vi "CalcVectors.vi"(8 "In/out":dbl, 9 "Up/down":dbl, 10 "Shoulder Degrees":dbl, 11 "Elbow Degrees":dbl) -> (2 "Shoulder Power":dbl, 3 "Elbow power":dbl)   [LabVIEW 2018]
panel:
  out "Theta C 2":dbl
  out "Theta b 2":dbl
  out "sin(b) 2":dbl
  out "sin(c) 2":dbl
  out "sin(b)":dbl
  out "sin(c)":dbl
  out "Theta C":dbl
  out "Theta b":dbl
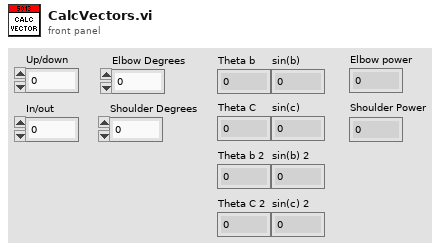
[diagram p1: front panel]
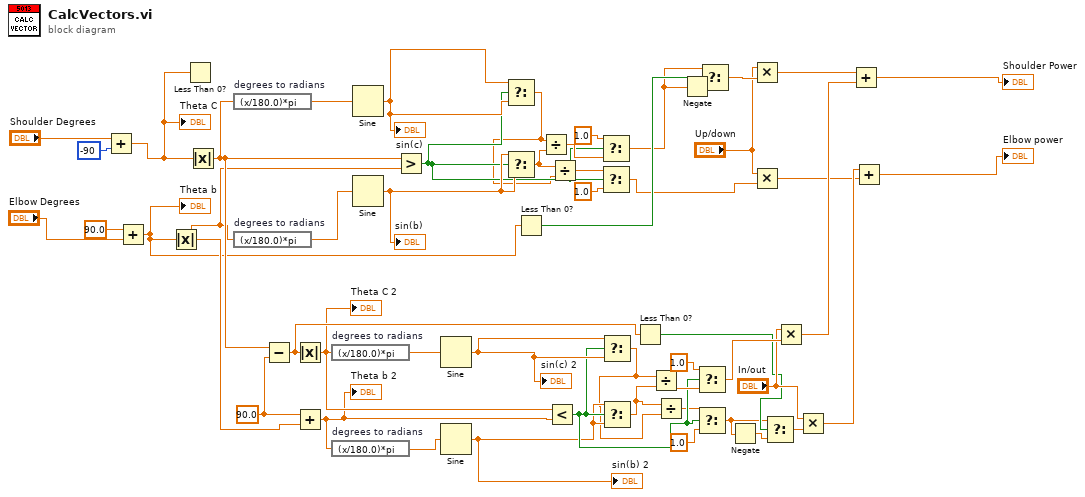
[diagram p0: block diagram]
diagram:
  w26 = 90.0 ("x")
  n1 = Add(x="Shoulder Degrees", y=-90) -> (x+y=w49:dbl)
  "Theta C" <- w49
  n2 = Add(x=90.0, y="Elbow Degrees") -> (x+y=w20:dbl)
  "Theta b" <- w20
  n3 = Absolute Value(x=w20) -> (abs(x)=w45:dbl)
  n4 = Less Than 0?(x=w49) -> ()  [unwired: 1 out]
  n5 = Absolute Value(x=w49) -> (abs(x)=w46:dbl)
  n6 = expression code="(x/180.0)*pi" "degrees to radians"(w46) -> (w43:dbl)
  n7 = expression code="(x/180.0)*pi" "degrees to radians"(w45) -> (w42:dbl)
  n8 = Subtract(x=w46, y=w26) -> (x-y=w25:dbl)
  n9 = Absolute Value(x=w25) -> (abs(x)=w18:dbl)
  "Theta C 2" <- w18
  n10 = Add(x=w26, y=w45) -> (x+y=w17:dbl)
  "Theta b 2" <- w17
  n11 = expression code="(x/180.0)*pi" "degrees to radians"(w18) -> (w33:dbl)
  n12 = expression code="(x/180.0)*pi" "degrees to radians"(w17) -> (w32:dbl)
  n13 = Sine(x=w43) -> (sin(x)=w41:dbl)
  "sin(c)" <- w41
  n14 = Sine(x=w42) -> (sin(x)=w40:dbl)
  "sin(b)" <- w40
  n15 = Greater?(x=w46, y=w45) -> (0:w34:bool)
  n16 = Sine(x=w33) -> (sin(x)=w31:dbl)
  "sin(c) 2" <- w31
  n17 = Sine(x=w32) -> (sin(x)=w21:dbl)
  "sin(b) 2" <- w21
  n18 = Select(t=w41, s=w34, f=w41) -> (s? t:f=w14:dbl)
  n19 = Select(t=w40, s=w34, f=w40) -> (s? t:f=w15:dbl)
  n20 = Less Than 0?(x=w20) -> (x < 0?=w13:bool)
  n21 = Divide(x=w14, y=w15) -> (x/y=w38:dbl)
  n22 = Less?(x=w18, y=w17) -> (x < y?=w24:bool)
  n23 = Divide(x=w15, y=w14) -> (x/y=w16:dbl)
  n24 = Select(t=1.0, s=w34, f=w38) -> (s? t:f=w7:dbl)
  n25 = Select(t=w16, s=w34, f=1.0) -> (s? t:f=w5:dbl)
  n26 = Select(t=w31, s=w24, f=w31) -> (s? t:f=w10:dbl)
  n27 = Select(t=w21, s=w24, f=w21) -> (s? t:f=w11:dbl)
  n28 = Less Than 0?(x=w25) -> (x < 0?=w3:bool)
  n29 = Divide(x=w10, y=w11) -> (x/y=w30:dbl)
  n30 = Divide(x=w11, y=w10) -> (x/y=w12:dbl)
  n31 = Negate(x=w7) -> (-x=w6:dbl)
  n32 = Select(t=1.0, s=w24, f=w30) -> (s? t:f=w28:dbl)
  n33 = Select(t=w12, s=w24, f=1.0) -> (s? t:f=w2:dbl)
  n34 = Select(t=w7, s=w13, f=w6) -> (s? t:f=w36:dbl)
  n35 = Negate(x=w2) -> (-x=w1:dbl)
  n36 = Multiply(x="Up/down", y=w36) -> (x*y=w8:dbl)
  n37 = Multiply(x="Up/down", y=w5) -> (x*y=w9:dbl)
  n38 = Select(t=w2, s=w3, f=w1) -> (s? t:f=w4:dbl)
  n39 = Multiply(x="In/out", y=w28) -> (x*y=w22:dbl)
  n40 = Multiply(x="In/out", y=w4) -> (x*y=w44:dbl)
  n41 = Add(x=w8, y=w22) -> (x+y=→"Shoulder Power":dbl)
  n42 = Add(x=w44, y=w9) -> (x+y=→"Elbow power":dbl)
